vi "ActPlaceCone.vi"() -> (3 "Done":bool)   [LabVIEW 2023]
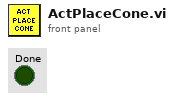
[diagram p1: front panel]
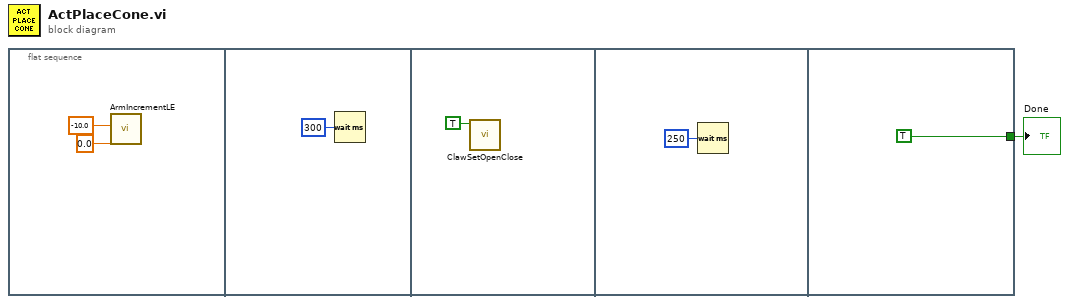
[diagram p0: block diagram]
diagram:
  n1 = flat-sequence {
    tunnel: [TRUE] -> w1
    frame #0 {
      n2 = call "ArmIncrementLE.vi"("AddE"=0.0, "AddL"=-10.0) -> ()  [unwired: 10 in]
    }
    frame #1 {
      n3 = Wait (ms)(milliseconds to wait=u32 300) -> ()  [unwired: 1 out]
    }
    frame #2 {
      n4 = call "ClawSetOpenClose.vi"("Open?"=TRUE) -> ()  [unwired: 11 in]
    }
    frame #3 {
      n5 = Wait (ms)(milliseconds to wait=u32 250) -> ()  [unwired: 1 out]
    }
    frame #4 {
    }
  }
  "Done" <- w1
